vi "Cycle Crossover.vi"(6 "Parent 2 Index":i32, 7 "Parent 1 Index":i32, 9 "Parent 2":T1, 10 "Parent 1":T1, 11 "OffSpring in":T1[](array[typedef])) -> (3 "OffSpring out":T1[](array[typedef]))   [LabVIEW 2013, in "GA.lvclass"]
uses:
  GA.lvclass
  Controls/Solution_GA.ctl
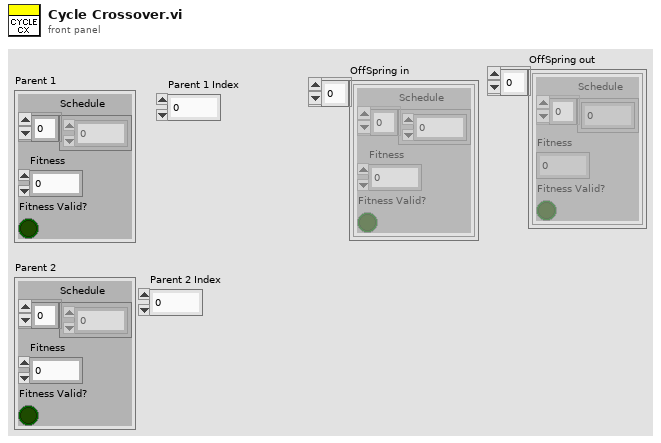
[diagram p1: front panel]
types:
  T1 = typedef "Solution_GA.ctl" = cluster{"Schedule":u16[], "Fitness":u16, "Fitness Valid?":bool}
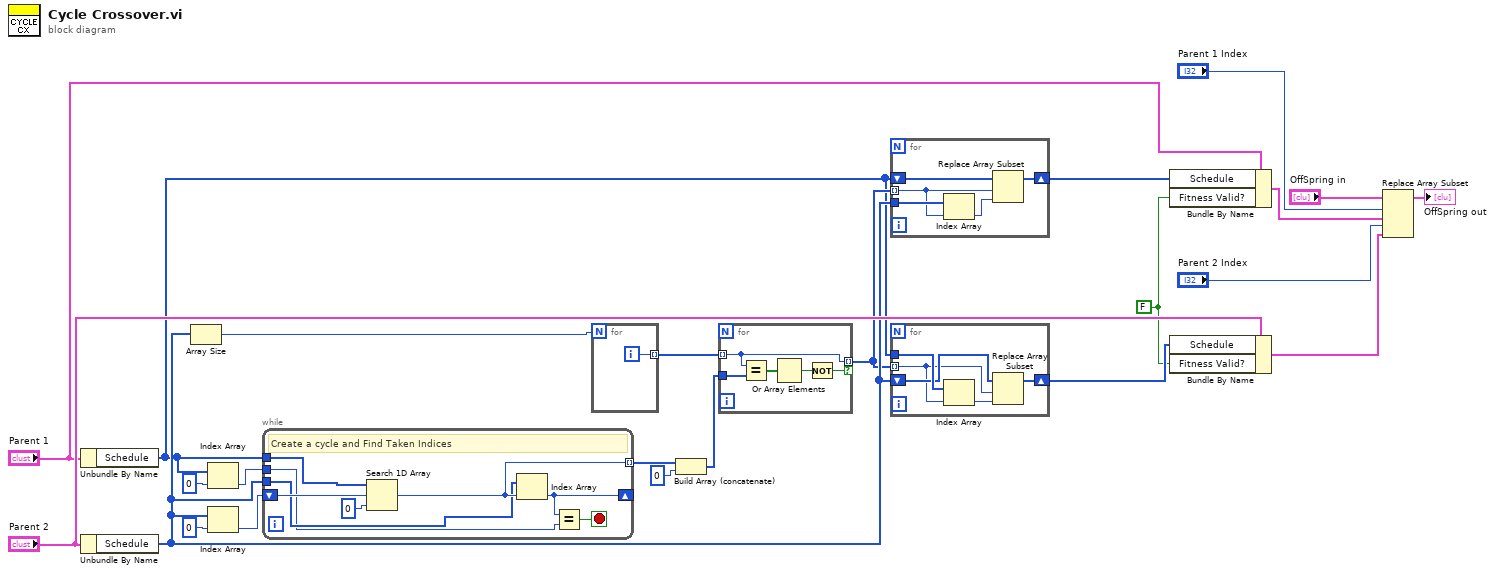
[diagram p0: block diagram]
diagram:
  w3 = FALSE ("Fitness Valid?")
  n1 = Unbundle By Name("Parent 1") -> ("Schedule"=w6:u16[])
  n2 = Unbundle By Name("Parent 2") -> ("Schedule"=w8:u16[])
  n3 = Array Size(array=w8) -> (size(s)=w11:i32)
  n4 = Index Array(array=w6, index=0) -> (element=w16:u16)
  n5 = Index Array(array=w8, index=0) -> (element=w14:u16)
  n6 = while {
    tunnel: w6 -> [w30]
    tunnel: w16 -> [w25]
    tunnel: [w31] -> w13 mode=indexing
    tunnel: w8 -> [w28]
    shift-right: [w26] -> _
    shift-left: w14 -> [w29]
    stop <- w24 stop-if-true
    # "Create a cycle and Find Taken Indices"
    n7 = Search 1D Array(1D array=w30, element=w29, start index (0)=0) -> (index of element=w31:i32)
    n8 = Index Array(array=w28, index=w31) -> (element=w26:u16)
    n9 = Equal?(x=w26, y=w25) -> (x = y?=w24:bool)
  }
  n10 = for {
    N: w11 -> [_]
    tunnel: [w32] -> w10 mode=indexing
    i -> [w32]
  }
  n11 = Build Array (concatenate)(w13, 0) -> (w9:i32[])
  n12 = for {
    tunnel: w10 -> [w37] mode=indexing
    tunnel: w9 -> [w36]
    tunnel: [w37] -> w7 mode=indexing if=w33
    n13 = Equal?(x=w37, y=w36) -> (x = y?=w35:bool[])
    n14 = Or Array Elements(Boolean array=w35) -> (logical OR=w34:bool)
    n15 = Not(x=w34) -> (.not. x?=w33:bool)
  }
  n16 = for {
    tunnel: w7 -> [w40] mode=indexing
    shift-right: [w38] -> w5
    shift-left: w6 -> [w41]
    tunnel: w8 -> [w42]
    n17 = Index Array(array=w42, index=w40) -> (element=w39:u16)
    n18 = Replace Array Subset(array=w41, new element=w39, index=w40) -> (w38:u16[])
  }
  n19 = for {
    tunnel: w7 -> [w45] mode=indexing
    shift-right: [w43] -> w4
    shift-left: w8 -> [w46]
    tunnel: w6 -> [w47]
    n20 = Index Array(array=w47, index=w45) -> (element=w44:u16)
    n21 = Replace Array Subset(array=w46, new element=w44, index=w45) -> (w43:u16[])
  }
  n22 = Bundle By Name(cluster="Parent 1", "Schedule"=w5, "Fitness Valid?"=w3) -> (w2:T1)
  n23 = Bundle By Name(cluster="Parent 2", "Schedule"=w4, "Fitness Valid?"=w3) -> (w1:T1)
  n24 = Replace Array Subset(array="OffSpring in", new element #1=w2, index #1="Parent 1 Index", new element #2=w1, index #2="Parent 2 Index") -> (→"OffSpring out":T1[])
